vi "PathPlanner_PathPlanner_Resolution.vi"() -> (3 "Resolution":dbl=0.004)   [LabVIEW 2019, in "PathPlanner.lvlib"]
uses:
  PathPlanner.lvlib
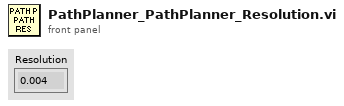
[diagram p1: front panel]
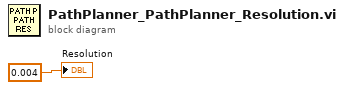
[diagram p0: block diagram]
diagram:
  "Resolution" <- 0.004
